vi "CaseStructure-Ver3-SlideControl.vi"() -> ()   [LabVIEW 2018]
panel:
  out "Less Than 7":bool
  out "Greater Than 7":bool
  out "Gauge":dbl(knob) scale=0.0..10.0
  in  "Slide":dbl(slide) scale=0.0..10.0
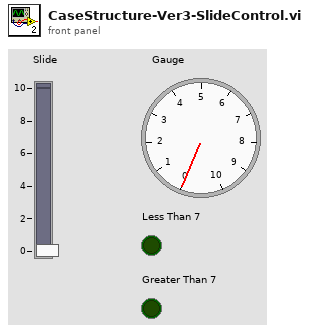
[diagram p1: front panel]
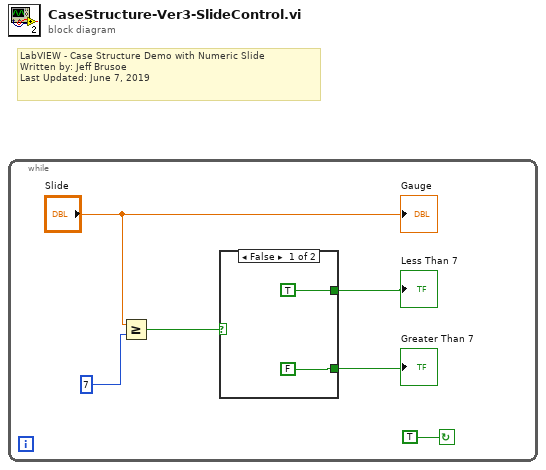
[diagram p0: block diagram]
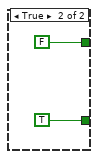
[diagram p2: hidden frame]
diagram:
  # "LabVIEW - Case Structure Demo with Numeric Slide\nWritten by: Jeff Brusoe\nLast Updated: June 7, 2019"
  n1 = while {
    stop <- TRUE continue-if-true
    n2 = Greater Or Equal?(x="Slide", y=7) -> (x >= y?=w1:bool)
    n3 = case shown="False" w1 {
      tunnel: [TRUE FALSE] -> w3
      tunnel: [FALSE TRUE] -> w2
      frame False {
      }
      frame True {
      }
    }
    "Greater Than 7" <- w2
    "Less Than 7" <- w3
    "Gauge" <- "Slide"
  }
